vi "PH_Sequencer.PC Write PSDB.vi"(0 "i ref in":refnum<vi>, 5 "error IO":errorcluster) -> (14 "i ref out":refnum<vi>, 19 "error out":errorcluster)   [LabVIEW 2014, in "PH_Sequencer.lvlib"]
doc: "This is the proc case which writes data to the PHELIX shot data base."
uses:
  PH_Sequencer.lvlib
  PH_PowerUnit_BaseClass/PH_PowerUnit_BaseClass.SM States.ctl
  PH_SystemInformation/PH_SystemInformationEnabling State.ctl
  PH_SystemInformation/PH_SystemInformation.lvlib
  PH_Common/PH_Common.lvlib
  PH_PSDBWriter/PH_PSDBWriter.lvlib
  PH_BeamlineInformation/PH_BeamlineInformation.lvlib
  PH_PowerUnit_BaseClass/PH_PowerUnit_BaseClass.lvlib
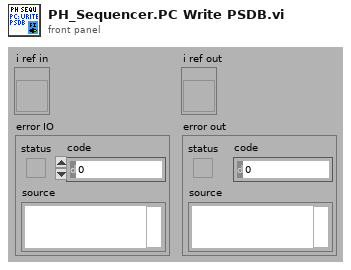
[diagram p1: front panel]
types:
  T1 = enum16{"Laser", "PreAmp", "MainAmp", "Exp 1", "Exp 2", "Exp 3", "Exp 4"}[]
  T2 = typedef "PH_BeamlineInformation.lvlib/PH_BeamlineInformation.i attribute.ctl" = cluster{"BL GUI Elements of Services":cluster{"Service Name":string, "GUI Elements":refnum<vi>[], "Status":i32}[], "Powermeters":T3, "Efficiency":T4, "Heads":T5[]}
  T3 = typedef "PH_BeamlineInformation.lvlib/PH_BeamlineInformation.Powermeter.ctl" = cluster{"ns FE":cluster{"GUI Ref":refnum<vi>, "Value":dbl}, "fs FE":cluster{"GUI Ref":refnum<vi>, "Value":dbl}, "PA":cluster{"GUI Ref":refnum<vi>, "Value":dbl}, "MA":cluster{"GUI Ref":refnum<vi>, "Value":dbl}, "Z6 green":cluster{"GUI Ref":refnum<vi>, "Value":dbl}, "Z6 IR":cluster{"GUI Ref":refnum<vi>, "Value":dbl}, "Z6 COS":cluster{"GUI Ref":refnum<vi>, "Value":dbl}}
  T4 = typedef "PH_BeamlineInformation.lvlib/PH_BeamlineInformation.Efficiency.ctl" = cluster{"PA Gain":cluster{"GUI Ref":refnum<vi>, "Value":dbl}, "MA Gain":cluster{"GUI Ref":refnum<vi>, "Value":dbl}, "Z6 green Conversion":cluster{"GUI Ref":refnum<vi>, "Value":dbl}, "Z6 Comp Losses":cluster{"GUI Ref":refnum<vi>, "Value":dbl}}
  T5 = typedef "PH_BeamlineInformation.lvlib/PH_BeamlineInformation.Head.ctl" = cluster{"PowerUnit":T6, "in use":cluster{"Value":bool, "GUI Ref":refnum<vi>, "linked":bool}, "voltage":cluster{"Value":dbl, "GUI Ref":refnum<vi>, "linked":bool}}
  T6 = typedef "PH_PP_Common.lvlib/PH_PP_Common.PUs.ctl" = enum16{"no Info", "PA-19mm-1", "PA-19mm-2", "PA-45mm-PILC", "PA-45mm-MAIN", "MA-PU-1", "MA-PU-2", "MA-PU-3", "MA-PU-4", "MA-PU-5", "MA-PU-6", "MA-FR", "MA-PILC", "PA-45mm-DP"}
  T7 = typedef "PH_Sequencer.lvlib/PH_Sequencer.i attribute.ctl" = cluster{"GUI Refs":cluster{"Main Off":refnum<vi>, "Fire":refnum<vi>, "Status":refnum<vi>, "Ready":refnum<vi>, "Waiting Time":refnum<vi>, "Timeout":refnum<vi>, "PPMA Ready":refnum<vi>, "Sequencer SM State":refnum<vi>, "PPPA Ready":refnum<vi>, "Calorimeter":refnum<vi>, "Beamline Ready":refnum<vi>, "Clear Beamline":refnum<vi>, "Linkage PPMA Rods":refnum<vi>, "Linkage Current PA":refnum<vi>, "Linkage Current MA":refnum<vi>, "Timing Ready":refnum<vi>, "State Timing":refnum<vi>, "Force Timing":refnum<vi>, "PSDB Shot Comment":refnum<vi>, "State PA Backreflection":refnum<vi>, "Beamline Z6 Ready":refnum<vi>, "Clear Z6 Beamline":refnum<vi>, "Sequence length":refnum<vi>, "Timing Mode":refnum<vi>, "Slow Trigger Settings":refnum<vi>, "Experiment Description":refnum<vi>, "State PSDB":refnum<vi>, "PSDB Ready":refnum<vi>, "Set PSDB Settings":refnum<vi>, "Get PSDB Info":refnum<vi>, "Take Snapshot":refnum<vi>, "Shottype":refnum<vi>, "Experiment":refnum<vi>, "Phase Frontends":refnum<vi>, "PP 45mm PILC in use":refnum<vi>}, "Status Info":cluster{"Machine Status":T8, "WaitingTime":i32, "Timeout":bool}, "Readyness":cluster{"Ready to shot":bool, "PPMA Ready":bool, "PPPA Ready":bool, "BL Ready":bool, "Timing Ready":bool, "BL Z6 Ready":bool, "PSDBReady":bool}, "Instancenames":cluster{"PPMA Rods":string, "PP Current Meas":string, "PH Beamline Chief":string, "PA Backrefl Meas":string, "Z6 Beamline Chief":string}, "Data to read":bool, "Calorimeter":cluster{"Instancename":string, "On":bool, "linked":bool}, "Linkage":cluster{"PPMA Rods":bool, "PP Current Meas":bool, "PHELIX Beamline Chief":bool, "PA Backrefl Meas":bool, "Z6 Beamline Chief":bool}, "Timing":cluster{"Instance":string, "linked":bool, "Status":T8, "Timing Mode":T9, "Slow Trigger Settings":T10, "Info available":cluster{"ext SlowTrigger":bool, "T2":bool, "Mode":bool, "Delay Slow Trigger":bool, "Phase FEs":bool}, "FE Phase":T11}, "Service ID R2S":i32, "PSDB":cluster{"Controller Instance":string, "Controller Status":T8, "Controller linked":bool, "Settings acknowledged":bool, "Current Experiment ID":i16, "Current Shot Type":i16, "Current Comment":string, "Remember Settings":bool, "Write 2 early":bool}, "PSDB Data":cluster{"Main Off?":bool, "Sequence Length":dbl, "Sequence startet":timestamp}, "6P 4Q Positions":cluster{"Instancename":string, "linked":bool, "Position":T12}[], "PUs":T13[]}
  T8 = typedef "PH_StatusHandler.lvlib/PH_StatusHandler.Status.ctl" = i16
  T9 = typedef "PH_Timing.lvlib/PH_Timing.Timing Mode.ctl" = cluster{"T2":i16, "Modeselector":enum32{"10 Hz", "0.5 Hz", "Shot"}}
  T10 = typedef "PH_Timing.lvlib/PH_Timing.Slow Trigger Settings.ctl" = cluster{"Delay":dbl, "externally triggered?":bool}
  T11 = typedef "PH_Timing.lvlib/PH_Timing.Phase FEs.ctl" = cluster{"Phase":dbl}
  T12 = typedef "PH_4_Pos_Selector.lvlib/PH_4_Pos_Selector.Position Selector.ctl" = u16
  T13 = typedef "PH_Sequencer.lvlib/PH_Sequencer.Head.ctl" = cluster{"PowerUnit":T6, "GUI Ref":refnum<vi>, "Information":T14, "linked?":bool, "GUI Ref Current Voltage":refnum<vi>}
  T14 = typedef "PH_Sequencer.lvlib/PH_Sequencer.PU Information.ctl" = cluster{"State":T8, "Waiting Time [s]":dbl, "PU State SM":T15, "PU Timeout SM":T15}
  T15 = typedef "PH_PowerUnit_BaseClass.lvlib/PH_PowerUnit_BaseClass.SM States.ctl" = enum16{".", "Stand by", "Switch PU on", "Configure", "Set Default Voltage", "Set STANDBY", "Set READY", "Wait for Shot Cmd", "Open Dump Rods", "Open Ross Relais", "Close Ross Relais", "Switch PSU on", "Switch PSU off", "Charge", "Switch GD Channel on", "Close Dump Rods", "Rods-TO", "RR-TO", "PSU-TO", "Trigger-TO"}
  T16 = typedef "PH_SystemInformation.lvlib/PH_SystemInformationEnabling State.ctl" = i32
  T17 = typedef "PH_PSDBWriter.lvlib/PH_PSDBWriter.Numeric dataset.ctl" = cluster{"name":string, "data":dbl, "unit":string}
  T18 = typedef "PH_PSDBWriter.lvlib/PH_PSDBWriter.Boolean dataset.ctl" = cluster{"name":string, "data":bool, "unit":string}
  T19 = typedef "PH_PSDBWriter.lvlib/PH_PSDBWriter.PSDB Dataset.ctl" = cluster{"Version":i32, "2D data Input":T20[], "Boolean Input":T18[], "Image Input":T22[], "Numeric Input":T17[], "String Input":T24[]}
  T20 = typedef "PH_PSDBWriter.lvlib/PH_PSDBWriter.2D dataset.ctl" = cluster{"name":string, "data":dbl[][], "axis description":T21}
  T21 = typedef "PSDB.lvlib/PSDB_AxisDescription.ctl" = cluster{"x axis label":string, "y axis label":string, "x axis unit":string, "y axis unit":string}
  T22 = typedef "PH_PSDBWriter.lvlib/PH_PSDBWriter.Image dataset.ctl" = cluster{"name":string, "data":T23, "unit":string}
  T23 = typedef "IMAQ Image.ctl" = refnum<image>
  T24 = typedef "PH_PSDBWriter.lvlib/PH_PSDBWriter.String dataset.ctl" = cluster{"name":string, "data":string, "unit":string}
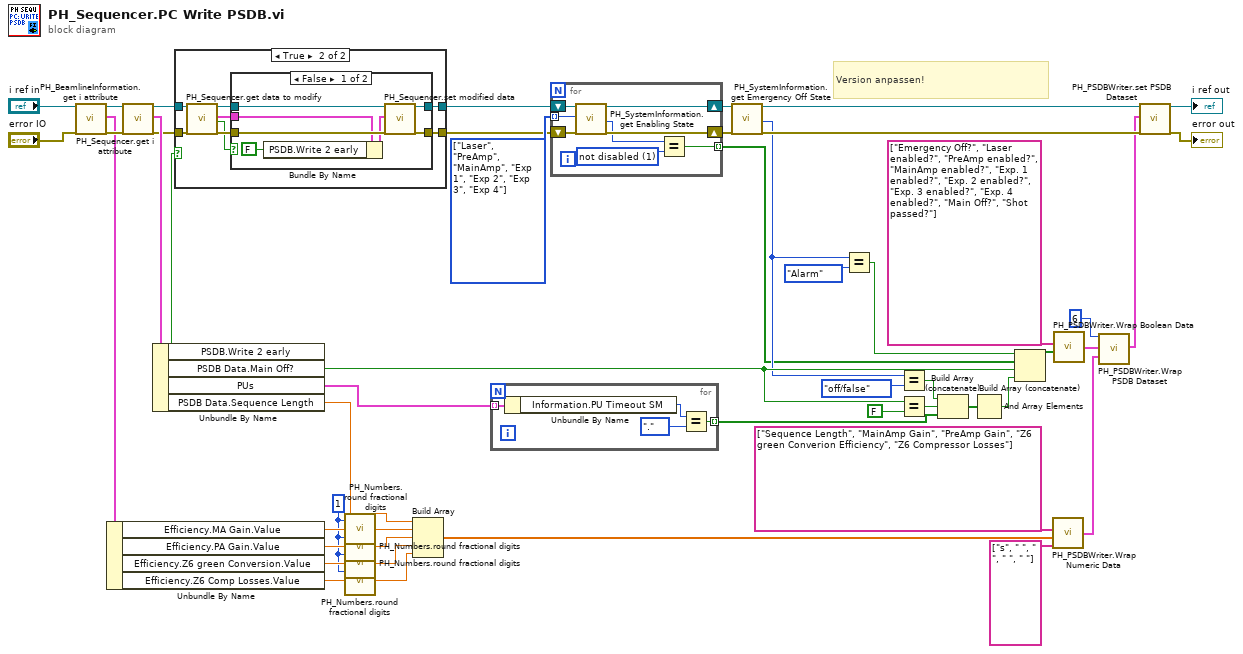
[diagram p0: block diagram]
diagram:
  w33 = T1 [enum."Laser", enum."PreAmp", enum."MainAmp", enum."Exp 1", enum."Exp 2", enum."Exp 3", enum."Exp 4"] items=["Laser", "PreAmp", "MainAmp", "Exp 1", "Exp 2", "Exp 3", "Exp 4"]
  w1 = i16 1 ("Position (1)")
  # "Version anpassen!"
  n1 = call "PH_BeamlineInformation.get i attribute.vi"("i ref in"="i ref in", "error in (no error)"="error IO") -> ("i ref out"=w12:refnum<vi>, "i attribute"=w11:T2, "error out"=w14:errorcluster)  [unwired: 15 in]
  n2 = Unbundle By Name(w11) -> ("Efficiency.MA Gain.Value"=w10:dbl, "Efficiency.PA Gain.Value"=w8:dbl, "Efficiency.Z6 green Conversion.Value"=w7:dbl, "Efficiency.Z6 Comp Losses.Value"=w6:dbl)
  n3 = call "PH_Sequencer.get i attribute.vi"("i ref in"=w12, "error in (no error)"=w14) -> ("i ref out"=w31:refnum<vi>, "i attribute"=w49:T7, "error out"=w29:errorcluster)  [unwired: 15 in]
  n4 = Unbundle By Name(w49) -> ("PSDB.Write 2 early"=w27:bool, "PSDB Data.Main Off?"=w43:bool, "PUs"=w9:T13[], "PSDB Data.Sequence Length"=w2:dbl)
  n5 = case shown="True" w27 {
    tunnel: w31 -> [w52 w56]
    tunnel: [w52 w55] -> w30
    tunnel: w29 -> [w51 w54]
    tunnel: [w51 w53] -> w28
    frame False {
    }
    frame True {
      n6 = call "PH_Sequencer.get data to modify.vi"("i ref in"=w56, "error in (no error)"=w54) -> ("i ref out"=w59:refnum<vi>, "i attribute"=w57:T7, "timed out"=w58:bool, "error out"=w60:errorcluster)  [unwired: 14 in]
      n7 = case shown="False" w58 {
        tunnel: w60 -> [w67 w68]
        tunnel: [w66 w68] -> w53
        tunnel: w59 -> [w65 w69]
        tunnel: [w64 w69] -> w55
        tunnel: w57 -> [w63 _]
        frame False {
          n8 = Bundle By Name(cluster=w63, "PSDB.Write 2 early"=FALSE) -> (w62:T7)
          n9 = call "PH_Sequencer.set modified data.vi"("i ref in"=w65, "i attribute"=w62, "error in (no error)"=w67) -> ("i ref out"=w64:refnum<vi>, "error out"=w66:errorcluster)  [unwired: 15 in]
        }
        frame True {
        }
      }
    }
  }
  n10 = call "PH_Numbers.round fractional digits.vi"("Input"=w10, "Position (1)"=w1) -> ("round Output"=w40:dbl)
  n11 = call "PH_Numbers.round fractional digits.vi"("Input"=w8, "Position (1)"=w1) -> ("round Output"=w5:dbl)
  n12 = call "PH_Numbers.round fractional digits.vi"("Input"=w7, "Position (1)"=w1) -> ("round Output"=w4:dbl)
  n13 = call "PH_Numbers.round fractional digits.vi"("Input"=w6, "Position (1)"=w1) -> ("round Output"=w3:dbl)
  n14 = Build Array(w2, w40, w5, w4, w3) -> (w19:dbl[])
  n15 = for {
    tunnel: w9 -> [w73] mode=indexing
    tunnel: [w70] -> w44 mode=indexing
    n16 = Unbundle By Name(w73) -> ("Information.PU Timeout SM"=w72:T15)
    n17 = Equal?(x=w72, y=PH_PowerUnit_BaseClass.SM_States.".") -> (x = y?=w70:bool)
  }
  n18 = for {
    shift-right: [w79] -> w34
    shift-left: w30 -> [w80]
    shift-right: [w77] -> w35
    shift-left: w28 -> [w81]
    tunnel: w33 -> [w78] mode=indexing
    tunnel: [w74] -> w32 mode=indexing
    w75 = T16 1 items=["no info", "not disabled", "disabled"] ("y")
    n19 = call "PH_SystemInformation.get Enabling State.vi"("i ref in"=w80, "Wanted State"=w78, "error in (no error)"=w81) -> ("i ref out"=w79:refnum<vi>, "Enabling State"=w76:T16, "error out"=w77:errorcluster)  [unwired: 14 in]
    n20 = Equal?(x=w76, y=w75) -> (x = y?=w74:bool)
  }
  n21 = call "PH_SystemInformation.get Emergency Off State.vi"("i ref in"=w34, "error in (no error)"=w35) -> ("i ref out"=w25:refnum<vi>, "Emergency Off State"=w36:enum16{"no info", "off/false", "Alarm"}, "error out"=w37:errorcluster)  [unwired: 15 in]
  n22 = Equal?(x=w36, y=enum16{"no info", "off/false", "Alarm"}."Alarm" ("Emergency Off State")) -> (x = y?=w42:bool)
  n23 = Equal?(x=w36, y=enum16{"no info", "off/false", "Alarm"}."off/false" ("Emergency Off State")) -> (x = y?=w41:bool)
  n24 = Equal?(x=w43, y=FALSE) -> (x = y?=w47:bool)
  n25 = Build Array (concatenate)(w41, w47, w44) -> (w46:bool[])
  n26 = And Array Elements(Boolean array=w46) -> (logical AND=w45:bool)
  n27 = Build Array (concatenate)(w42, w32, w43, w45) -> (w22:bool[])
  n28 = call "PH_PSDBWriter.Wrap Numeric Data.vi"("Unit Array"=string[] ["s", " ", " ", " ", " "], "Data Array"=w19, "Name Array"=string[] ["Sequence Length", "MainAmp Gain", "PreAmp Gain", "Z6 green Converion Efficiency", "Z6 Compressor Losses"]) -> ("PSDB Numeric Data Array"=w17:T17[])  [unwired: 1 in]
  n29 = call "PH_PSDBWriter.Wrap Boolean Data.vi"("Data Array"=w22, "Name Array"=string[] ["Emergency Off?", "Laser enabled?", "PreAmp enabled?", "MainAmp enabled?", "Exp. 1 enabled?", "Exp. 2 enabled?", "Exp. 3 enabled?", "Exp. 4 enabled?", "Main Off?", "Shot passed?"]) -> ("PSDB Boolean Data Array"=w21:T18[])  [unwired: 2 in]
  n30 = call "PH_PSDBWriter.Wrap PSDB Dataset.vi"("Version"=6, "Boolean Input"=w21, "Numeric Input"=w17) -> ("PSDB Dataset"=w16:T19)  [unwired: 16 in]
  n31 = call "PH_PSDBWriter.set PSDB Dataset.vi"("VI in"=w25, "PSDB Dataset"=w16, "error in (no error)"=w37) -> ("VI out"=→"i ref out":refnum<vi>, "error out"=→"error out":errorcluster)  [unwired: 15 in]
